vi "Facade 1.vi"(0 "Data In":T5, 2 "Display State In":T3, 3 "Container State":T4) -> (6 "Data Out":T5, 7 "Display State Out":T3, 8 "Action":T2)   [LabVIEW 2023, in "System Button.xctl"]
uses:
  System Button.xctl
  Data 1.ctl
  <vilib>/_xctls/Container State.ctl
  State 1.ctl
  <vilib>/_xctls/Action.ctl
  <vilib>/_xctls/XControlSupport.lvlib
panel:
  in  "System Cluster":T1
  in  "Button":bool caption="Boolean"
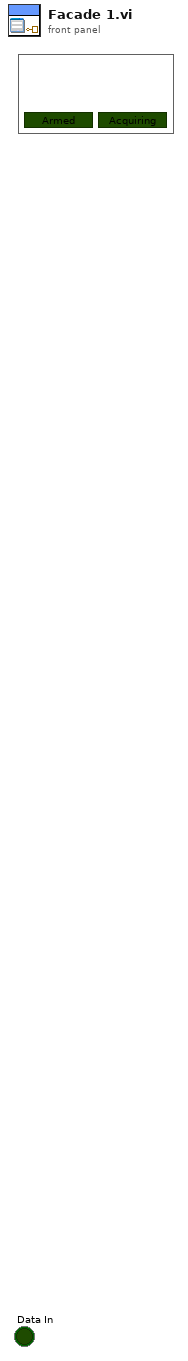
[diagram p1: front panel]
types:
  T1 = cluster{"Armed":bool, "Acquiring":bool, "System Type":string, "System ID":string, "System ID Big":string}
  T2 = typedef "XControlSupport.lvlib/Action.ctl" = cluster{"Data Changed?":bool, "State Changed?":bool, "Action Name":string}
  T3 = typedef "System Button.xctl/State 1.ctl" = cluster{"Armed":bool, "Acquiring":bool, "System Type":string, "System ID":string, "System ID Big":string}
  T4 = typedef "XControlSupport.lvlib/Container State.ctl" = cluster{"Indicator?":bool, "Run Mode?":bool, " Refnum":refnum<vi>}
  T5 = typedef "System Button.xctl/Data 1.ctl" = bool
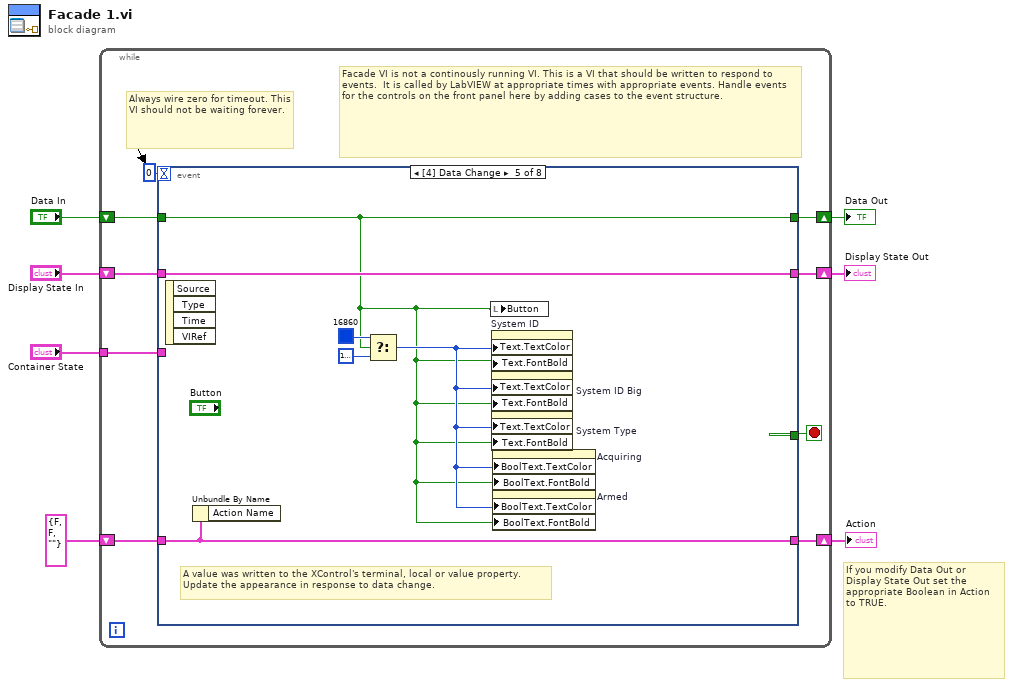
[diagram p0: block diagram]
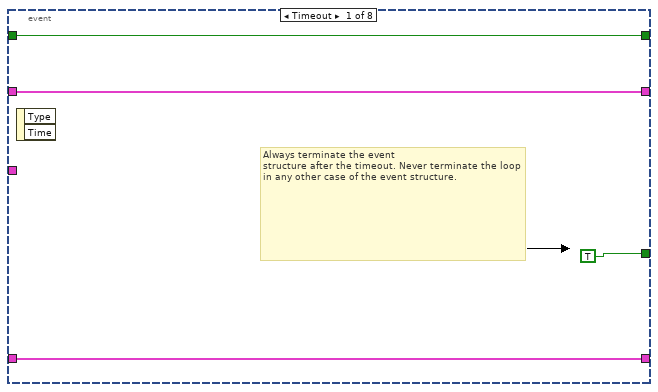
[diagram p2: hidden frame]
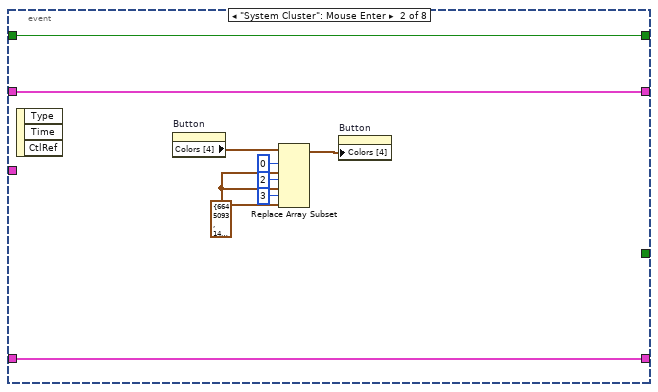
[diagram p3: hidden frame]
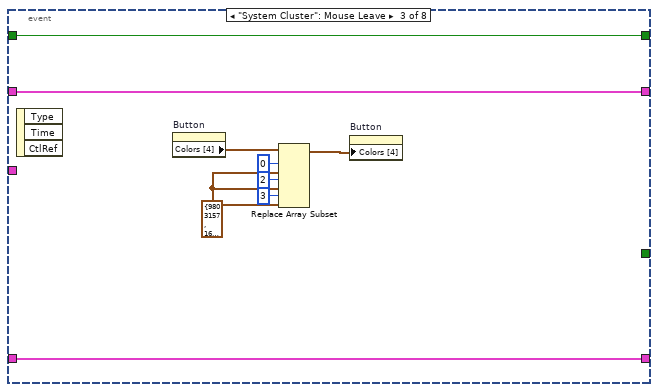
[diagram p4: hidden frame]
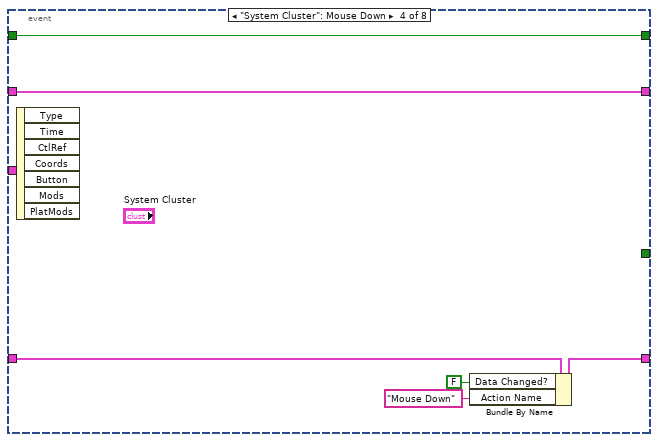
[diagram p5: hidden frame]
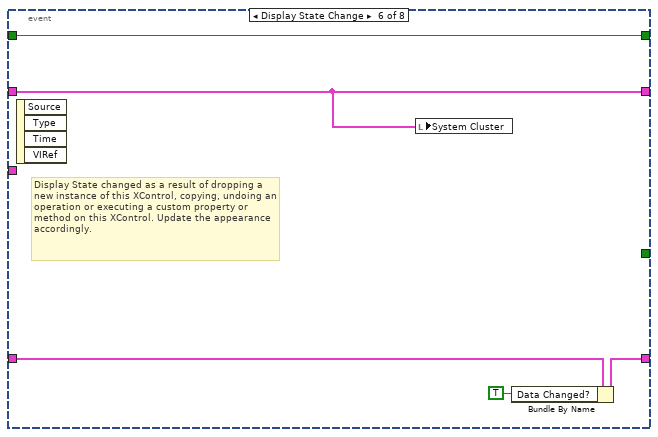
[diagram p6: hidden frame]
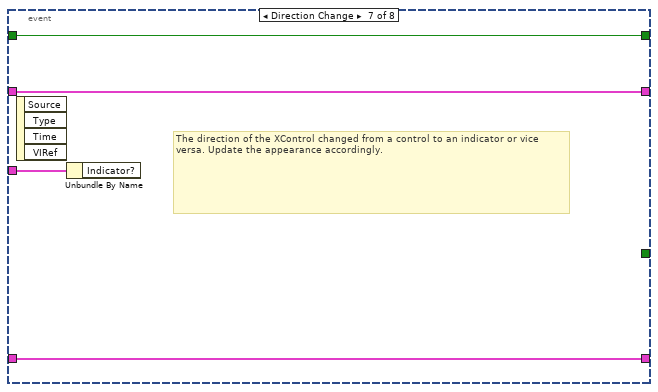
[diagram p7: hidden frame]
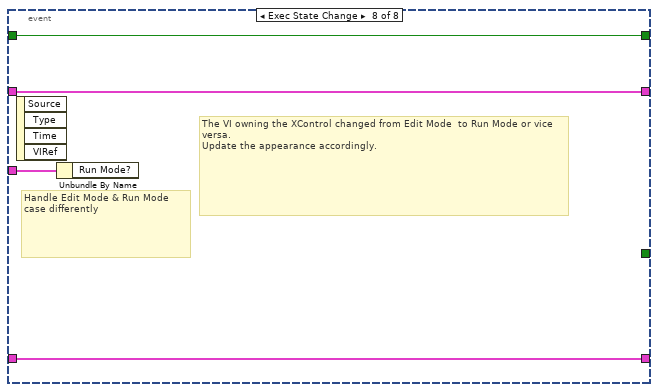
[diagram p8: hidden frame]
diagram:
  # "If you modify Data Out or\nDisplay State Out set the\nappropriate Boolean in Action\nto TRUE."
  n1 = while {
    shift-right: [w15] -> w4
    shift-left: "Display State In" -> [w16]
    tunnel: "Container State" -> [w12]
    shift-right: [w10] -> w7
    shift-left: "Data In" -> [w11]
    shift-right: [w8] -> w2
    shift-left: T2 {"Data Changed?"=FALSE, "State Changed?"=FALSE, "Action Name"=""} ("Action") -> [w9]
    stop <- w14 stop-if-true
    # "Facade VI is not a continously running VI. This is a VI that should be written to respond to events.  It is called by LabVIEW at appropriate times with appropriate events. Handle events for the controls on the front panel here by adding cases to the event structure."
    # "Always wire zero for timeout. This\nVI should not be waiting forever."
    n2 = event shown="[4] Data Change" {
      selector: _ -> [_ _ _ _ _ _ _ _]
      dyn-events: _ -> [_ _ _ _ _ _ _ _]
      timeout: 0 -> [_ _ _ _ _ _ _ _]
      tunnel: w16 -> [w18 w28 w37 w41 w50 w51 w58 w62]
      tunnel: [w18 w28 w37 w41 w50 w51 w58 w62] -> w15
      tunnel: [TRUE _ _ _ _ _ _ _] -> w14
      tunnel: w12 -> [_ _ _ _ _ _ w59 w63]
      tunnel: w11 -> [w17 w29 w38 w40 w45 w52 w57 w61]
      tunnel: [w17 w29 w38 w40 w45 w52 w57 w61] -> w10
      tunnel: [w19 w27 w36 w43 w46 w54 w56 w60] -> w8
      tunnel: w9 -> [w19 w27 w36 w44 w46 w55 w56 w60]
      event Timeout {
        # "Always terminate the event\nstructure after the timeout. Never terminate the loop in any other case of the event structure."
        n3 = event-data() -> ()  [unwired: 1 in, 2 out]
      }
      event "System Cluster": Mouse Enter {
        w21 = cluster{u32, u32} {6645093, 14606046}
        n4 = event-data() -> ()  [unwired: 1 in, 3 out]
        n5 = property on="Button" class="Bool (strict)"() -> ("Colors [4]"=w26:cluster{u32, u32}[])  [unwired: 2 in, 2 out]
        n6 = Replace Array Subset(array=w26, new element #1=w21, index #1=0 ("index"), new element #2=w21, index #2=2 ("index"), new element #3=w21, index #3=3 ("index")) -> (w25:cluster{u32, u32}[])
        n7 = property on="Button" class="Bool (strict)"("Colors [4]"=w25) -> ()  [unwired: 2 in, 2 out]
      }
      event "System Cluster": Mouse Leave {
        w30 = cluster{u32, u32} {9803157, 16777215}
        n8 = event-data() -> ()  [unwired: 1 in, 3 out]
        n9 = property on="Button" class="Bool (strict)"() -> ("Colors [4]"=w35:cluster{u32, u32}[])  [unwired: 2 in, 2 out]
        n10 = Replace Array Subset(array=w35, new element #1=w30, index #1=0 ("index"), new element #2=w30, index #2=2 ("index"), new element #3=w30, index #3=3 ("index")) -> (w34:cluster{u32, u32}[])
        n11 = property on="Button" class="Bool (strict)"("Colors [4]"=w34) -> ()  [unwired: 2 in, 2 out]
      }
      event "System Cluster": Mouse Down {
        n12 = event-data() -> ()  [unwired: 1 in, 7 out]
        n13 = Bundle By Name(cluster=w44, "Data Changed?"=FALSE, "Action Name"="Mouse Down") -> (w43:T2)
      }
      event Data Change {
        # "A value was written to the XControl's terminal, local or value property.\nUpdate the appearance in response to data change."
        n14 = event-data() -> ()  [unwired: 1 in, 4 out]
        n15 = Unbundle By Name(w46) -> ()  [unwired: 1 out]
        n16 = Select(t=u32 16860, s=w45, f=u32 16777222) -> (s? t:f=w48:u32)
        n17 = local write "Button"(w45) -> ()
        n18 = property on="System ID" class="Str"("Text.TextColor"=w48, "Text.FontBold"=w45) -> ()  [unwired: 2 in, 2 out]
        n19 = property on="System ID Big" class="Str"("Text.TextColor"=w48, "Text.FontBold"=w45) -> ()  [unwired: 2 in, 2 out]
        n20 = property on="System Type" class="Str"("Text.TextColor"=w48, "Text.FontBold"=w45) -> ()  [unwired: 2 in, 2 out]
        n21 = property on="Acquiring" class="Bool (strict)"("BoolText.TextColor"=w48, "BoolText.FontBold"=w45) -> ()  [unwired: 2 in, 2 out]
        n22 = property on="Armed" class="Bool (strict)"("BoolText.TextColor"=w48, "BoolText.FontBold"=w45) -> ()  [unwired: 2 in, 2 out]
      }
      event Display State Change {
        # "Display State changed as a result of dropping a new instance of this XControl, copying, undoing an operation or executing a custom property or method on this XControl. Update the appearance accordingly."
        n23 = event-data() -> ()  [unwired: 1 in, 4 out]
        n24 = local write "System Cluster"(w51) -> ()
        n25 = Bundle By Name(cluster=w55, "Data Changed?"=TRUE) -> (w54:T2)
      }
      event Direction Change {
        # "The direction of the XControl changed from a control to an indicator or vice versa. Update the appearance accordingly."
        n26 = event-data() -> ()  [unwired: 1 in, 4 out]
        n27 = Unbundle By Name(w59) -> ()  [unwired: 1 out]
      }
      event Exec State Change {
        # "The VI owning the XControl changed from Edit Mode  to Run Mode or vice versa.\nUpdate the appearance accordingly."
        # "Handle Edit Mode & Run Mode\ncase differently"
        n28 = event-data() -> ()  [unwired: 1 in, 4 out]
        n29 = Unbundle By Name(w63) -> ()  [unwired: 1 out]
      }
    }
  }
  "Display State Out" <- w4
  "Data Out" <- w7
  "Action" <- w2
